vi "Round Sequence Time.vi"(8 "error in":errorcluster, 11 "Input Sequence":T3(array[cluster])) -> (0 "error out":errorcluster, 3 "Sequence After Round":T3(array[cluster]))   [LabVIEW 2020]
uses:
  Labview Library/Libraries/HW_LMMR_ASG8100/LMMR ASG/Loop Config.ctl
  Labview Library/Libraries/HW_LMMR_ASG8100/LMMR ASG/Loop Code.ctl
  <vilib>/Utility/error.llb/DialogType.ctl
  Labview Library/Libraries/HW_LMMR_ASG8100/LMMR ASG/Loop XControl.xctl
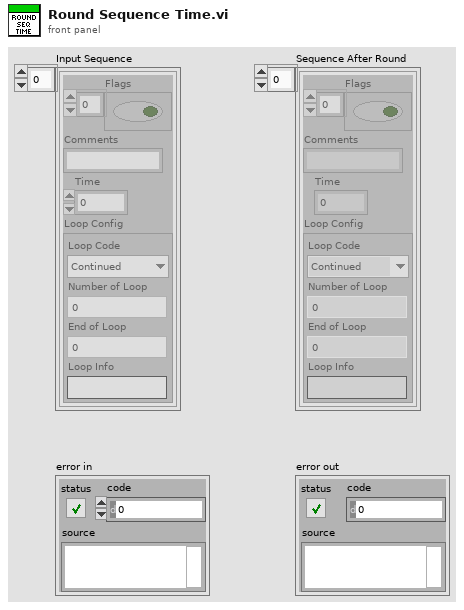
[diagram p1: front panel]
types:
  T1 = typedef "Loop XControl.xctl/Loop Config.ctl" = cluster{"Loop Code":T2, "Number of Loop":i32, "End of Loop":dbl, "Loop Info":string}
  T2 = typedef "Loop XControl.xctl/Loop Code.ctl" = enum16{"Continued", "Loop", "End Loop"}
  T3 = cluster{"Flags":bool[], "Comments":string, "Time":dbl, "Loop Config":T1}[]
  T4 = typedef "DialogType.ctl" = u16
  T5 = cluster{"Flags":bool[], "Comments":string, "Time":dbl, "Loop Config":T1}
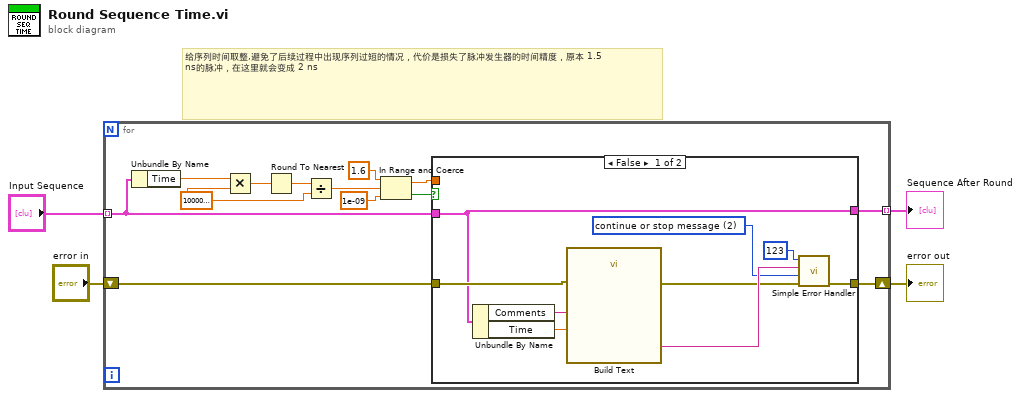
[diagram p0: block diagram]
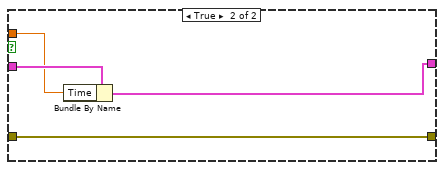
[diagram p2: hidden frame]
diagram:
  # "给序列时间取整,避免了后续过程中出现序列过短的情况，代价是损失了脉冲发生器的时间精度，原本 1.5 ns的脉冲，在这里就会变成 2 ns"
  n1 = for {
    tunnel: "Input Sequence" -> [w9] mode=indexing
    shift-right: [w8] -> w3
    shift-left: "error in" -> [w7]
    tunnel: [w5] -> w4 mode=indexing
    w14 = 1000000000.0 ("Numeric")
    n2 = Unbundle By Name(w9) -> ("Time"=w17:dbl)
    n3 = Multiply(x=w17, y=w14) -> (x*y=w16:dbl)
    n4 = Round To Nearest(number=w16) -> (nearest integer value=w15:dbl)
    n5 = Divide(x=w15, y=w14) -> (x/y=w13:dbl)
    n6 = In Range and Coerce(upper limit=1.6 ("lower limit"), x=w13, lower limit=1e-09) -> (coerced(x)=w6:dbl, In Range?=w10:bool)
    n7 = case shown="False" w10 {
      tunnel: w9 -> [w18 w29]
      tunnel: [w22 w30] -> w8
      tunnel: w7 -> [w21 w30]
      tunnel: w6 -> [_ w28]
      tunnel: [w18 w27] -> w5
      frame False {
        w19 = T4 2 items=["no dialog", "OK message", "continue or stop message", "OK message + warnings", "continue/stop + warnings"] ("type of dialog (OK msg:1)")
        n8 = Unbundle By Name(w18) -> ("Comments"=w25:string, "Time"=w26:dbl)
        n9 = call "Build Text"("name"=w25, "time"=w26, "error in (no error)"=w21) -> ("Result"=w24:string, "error out"=w20:errorcluster)  [unwired: 11 in]
        n10 = call <vilib>:"Simple Error Handler.vi"("error code (no error:0)"=123, "error source (\" \")"=w24, "type of dialog (OK msg:1)"=w19, "error in (no error)"=w20) -> ("error out"=w22:errorcluster)  [unwired: 1 in, 4 out]
      }
      frame True {
        n11 = Bundle By Name(cluster=w29, "Time"=w28) -> (w27:T5)
      }
    }
  }
  "Sequence After Round" <- w4
  "error out" <- w3
